vi "CSMOMgr-Duplication Check.vi"(8 "Error in":errorcluster caption="Error in (no error)", 10 "Queue Name":string, 11 "CSMOMgr":T1) -> (0 "Error out":errorcluster, 3 "CSMOMgr out":T1)   [LabVIEW 2020, in "Communicable State Machine.lvlib"]
uses:
  Communicable State Machine.lvlib
  Def-CSMOMgr.ctl
  _CSMObj.ctl
  _CSM_MODE.ctl
  Priority Queue.lvclass
  _CSMObj-Data.ctl
  _CSM Status Change Event Data.ctl
  _CSMObj-ModeData.ctl
  Priority Queue.lvclass/Priority Queue.ctl
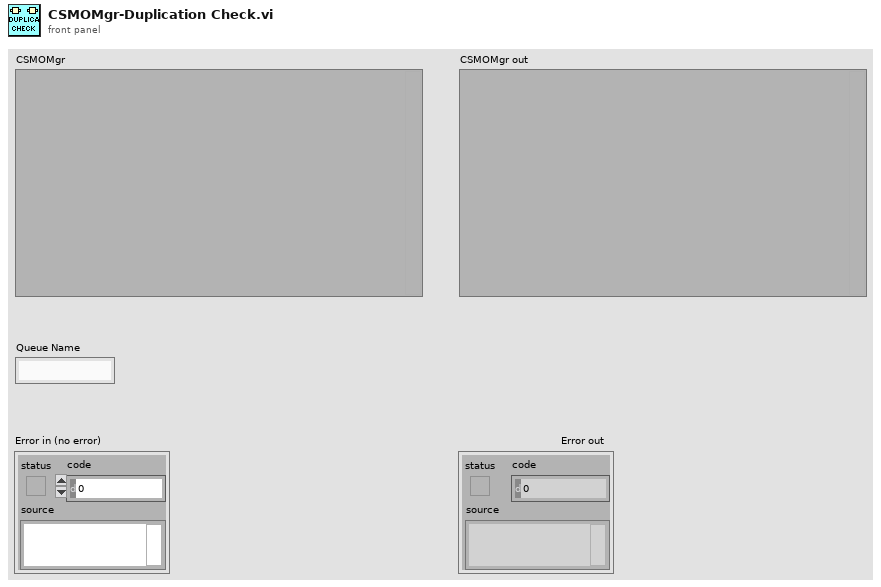
[diagram p1: front panel]
types:
  T1 = typedef "Communicable State Machine.lvlib/Def-CSMOMgr.ctl" = variant
  T2 = typedef "Communicable State Machine.lvlib/_CSMObj.ctl" = cluster{"Requested Name":string, "Module Name":string, "Mode":T3, "Queue":refnum<class "Priority Queue.lvclass">, "CSM-Data":refnum<data-value>, "User Event":refnum<user-event>, "Status Change Event":refnum<user-event>, "Allowed Messages":string[], "Mode-Data":refnum<data-value>, "Group Name":string, "Exit Event":refnum<user-event>}
  T3 = typedef "Communicable State Machine.lvlib/_CSM_MODE.ctl" = enum16{"Not Exist", "Stand Alone", "CSM", "Worker Agent", "Worker", "Chain", "Chain Node"}
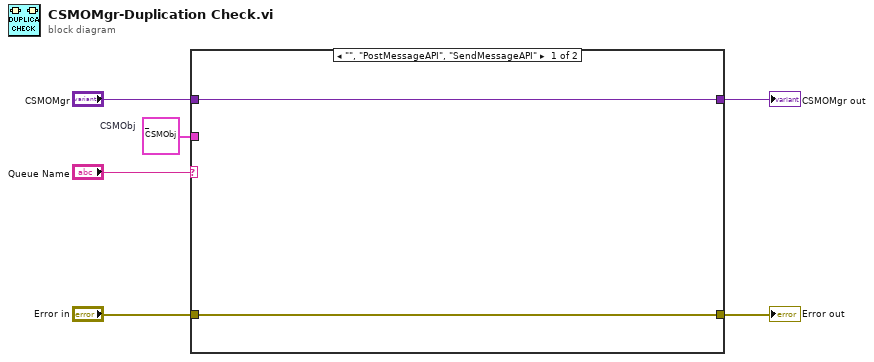
[diagram p0: block diagram]
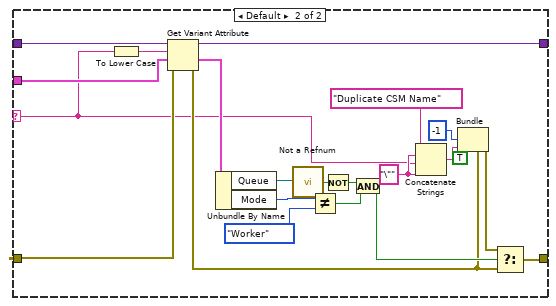
[diagram p2: hidden frame]
diagram:
  w1 = T2 {"Requested Name"="", "Module Name"="", "Mode"=enum."Stand Alone", "Queue"=refnum, "CSM-Data"=refnum, "User Event"=refnum, "Status Change Event"=refnum, "Allowed Messages"=[], "Mode-Data"=refnum, "Group Name"="", "Exit Event"=refnum}  # CSMObj
  n1 = case shown="\"\", \"PostMessageAPI\", \"SendMessageAPI\"" "Queue Name" {
    selector: "Queue Name" -> [_ w10]
    tunnel: [w7 w30] -> w3
    tunnel: "Error in" -> [w7 w13]
    tunnel: "CSMOMgr" -> [w8 w15]
    tunnel: [w8 w14] -> w2
    tunnel: w1 -> [_ w11]
    frame "", "PostMessageAPI", "SendMessageAPI" {
    }
    frame Default {
      w24 = "\"" ("string")
      n2 = To Lower Case(string=w10) -> (all lower case string=w9:string)
      n3 = Get Variant Attribute(Variant=w15, name=w9, default value (empty Variant)=w11, error in=w13) -> (duplicate Variant=w14:variant, value=w17:T2, error out=w12:errorcluster)  [unwired: 1 out]
      n4 = Unbundle By Name(w17) -> ("Queue"=w18:refnum<class "Priority Queue.lvclass">, "Mode"=w21:T3)
      n5 = call "Not a Refnum.vi"("Priority Queue.lvclass"=w18) -> ("NaN/Path/Refnum?"=w19:bool)  [unwired: 4 in]
      n6 = Not Equal?(x=w21, y=_CSM_MODE."Worker") -> (x != y?=w23:bool)
      n7 = Not(x=w19) -> (.not. x?=w20:bool)
      n8 = And(x=w20, y=w23) -> (x .and. y?=w16:bool)
      n9 = Concatenate Strings("Duplicate CSM Name" ("String to Prepend to source (\"\")"), w24, w10, w24) -> (w25:string)
      n10 = Bundle(cluster=w12, "status"=TRUE, "code"=-1, "source"=w25) -> (w29:errorcluster)
      n11 = Select(t=w29, s=w16, f=w12) -> (s? t:f=w30:errorcluster)
    }
  }
  "Error out" <- w3
  "CSMOMgr out" <- w2
